vi "Auto.vi"() -> ()   [LabVIEW 2020]
uses:
  Global_Variable/Global.vi
  Global_Variable/A180648.vi
  Global_Variable/System_Conf.vi
  <userlib>/_MGI/1D Array/MGI Running Average/MGI Running Average(DBL).vi
  <userlib>/_MGI/1D Array/MGI Running Average/MGI Running Average(SGL).vi
  Libraries/S7/S7.lvlib
panel:
  out "工位三开始1":u32
  out "工位三开始":u32
  out "工位2开始":u32
  out "用户事件输出":refnum<user-event>
  out "磨合正向初始化":bool
  out "工位三开始计时1":bool
  out "产品变更_Event":refnum<user-event>
  out "NVH":bool=TRUE
  out "T1+T2":dbl
  out "T2":dbl
  out "T1":dbl
  out "吸收电流":sgl
  out "输出扭矩(大)":sgl
  out "输入扭矩":sgl
  out "力特性逆向去程":bool
  out "力特性正向去程":bool
  out "力特性逆向回程":bool
  out "力特性正向回程":bool
  out "工位三开始计时":bool
  out "工位二开始计时":bool
  out "功能正向初始化":bool
  out "功能逆向初始化":bool
  out "空载逆向初始化":bool
  out "空载正向初始化":bool
  out "试验项目":T1(tab)
  out "压装曲线":cluster{dbl[], dbl[]}[](graph)
  out "侧铆曲线":cluster{dbl[], dbl[]}[](graph)
  out "0°曲线":cluster{dbl[], dbl[]}[](graph)
  out "45°曲线":cluster{dbl[], dbl[]}[](graph)
  out "力特性试验":cluster{dbl[], dbl[]}[](graph)
  out "功能试验":cluster{dbl[], dbl[]}[](graph)
  out "电流特性试验":cluster{dbl[], dbl[]}[](graph)
  out "逆向空载试验":cluster{dbl[], dbl[]}[](graph)
  out "磨合":cluster{dbl[], dbl[]}[](graph)
  in  "判定结果":bool[][](array[boolean])=[[TRUE]]
  in  "STEP":string
  # "车速0"
  # "车速1"
  # "车速2"
  # "车速3"
  # "车速4"
  # "车速5"
  # "车速0"
  # "车速1"
  # "车速2"
  # "车速3"
  # "车速4"
  # "车速5"
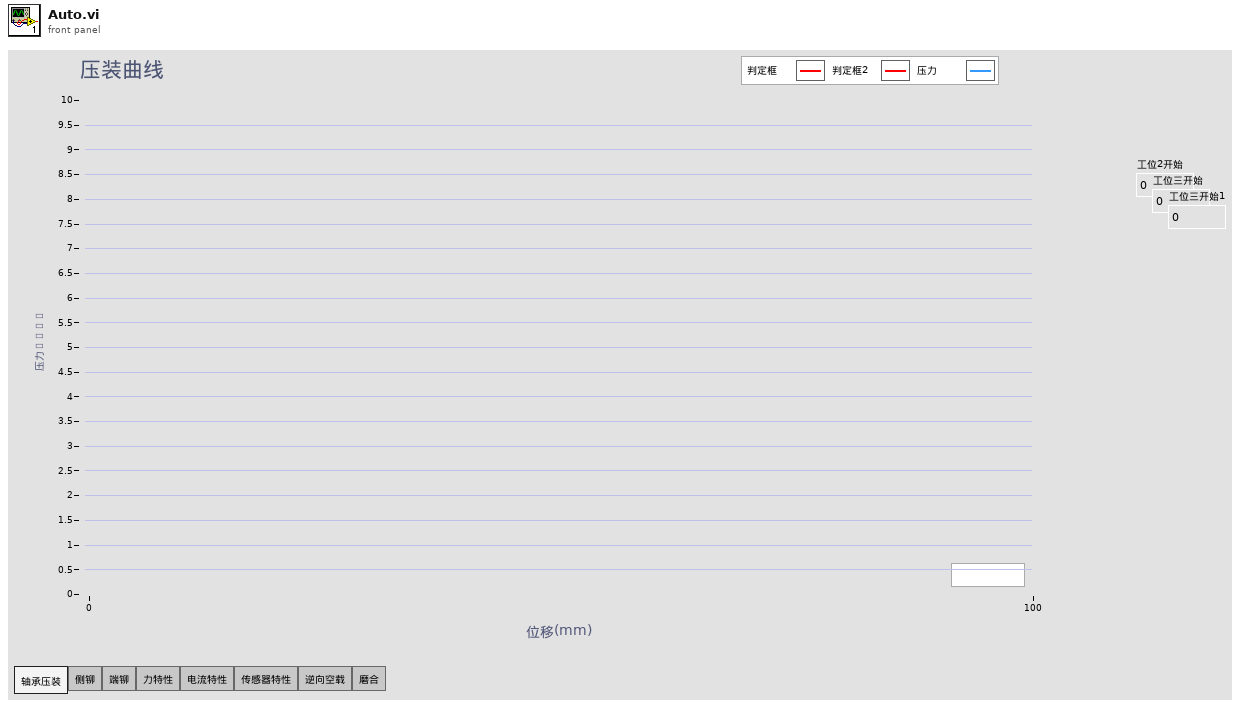
[diagram p1: front panel]
types:
  T1 = enum32{"轴承压装", "侧铆", "端铆", "力特性", "电流特性", "传感器特性", "逆向空载", "磨合"}
  T2 = enum32{"Invalid", "Standard", "Closed", "Hidden", "Minimized", "Maximized"}
  T3 = typedef "lveventtype.ctl" = enum32{"Null", "Timeout", "Annotation Menu Selection", "Annotation Menu Selection?", "App Instance Close", "App Instance Close?", "Autoscale Range Change", "Bookmark Info Change", "Cell Edit", "Cell Edit?", "Cursor Grab", "Cursor Grab?", "Cursor Menu Selection", "Cursor Menu Selection?", "Cursor Move", "Cursor Release", "Data Change", "Direction Change", "Display State Change", "Drag Ended", "Drag Enter", "Drag Leave", "Drag Over", "Drag Source Update", "Drag Starting", "Drag Starting?", "Drop", "Exec State Change", "Key Down", "Key Down?", "Key Repeat", "Key Repeat?", "Key Up", "Listbox Double Click", "Menu Activation?", "Menu Selection (App)", "Menu Selection? (App)", "Menu Selection (User)", "Mouse Down", "Mouse Down?", "Mouse Enter", "Mouse Leave", "Mouse Move", "Mouse Up", "Mouse Wheel", "NI Security User Change (App)", "Pane Size", "Panel Close", "Panel Close?", "Panel Resize", "Plot Attribute Change", "Scale Range Change", "Shortcut Menu Activation?", "Shortcut Menu Selection (App)", "Shortcut Menu Selection? (App)", "Shortcut Menu Selection (User)", "Tree Double Click", "Tree Drag", "Tree Drag?", "Tree Drop", "Tree Drop?", "Tree Item Close", "Tree Item Close?", "Tree Item Open", "Tree Item Open?", "User Event", "Value Change"}
  T4 = typedef "LVPoint32TypeDef.ctl" = cluster{"Horizontal":i32, "Vertical":i32}
  T5 = cluster{"输入轴扭矩":dbl, "输出轴扭矩小量程":dbl, "输出轴扭矩大量程":dbl}
  T6 = typedef "System_conf.ctl" = cluster{"空载滤波":bool, "逆向空载滤波":bool, "空载扭矩系数":dbl, "逆向空载扭矩系数":dbl}
  T7 = cluster{"1位移":cluster{"单位":string, "下限":dbl, "上限":dbl}, "1压力":cluster{"单位":string, "下限":dbl, "上限":dbl}, "2位移":cluster{"单位":string, "下限":dbl, "上限":dbl}, "2压力":cluster{"单位":string, "下限":dbl, "上限":dbl}}
  T8 = cluster{"第一段位移区间最大压力":cluster{"单位":string, "下限":dbl, "上限":dbl}, "第一段位移区间最小压力":cluster{"单位":string, "下限":dbl, "上限":dbl}, "第二段位移区间最大压力":cluster{"单位":string, "下限":dbl, "上限":dbl}, "第二段位移区间最小压力":cluster{"单位":string, "下限":dbl, "上限":dbl}, "压装最终位移":cluster{"单位":string, "下限":dbl, "上限":dbl}}
  T9 = cluster{"侧铆最大压力":cluster{"单位":string, "下限":dbl, "上限":dbl}}
  T10 = cluster{"端铆最大压力":cluster{"单位":string, "下限":dbl, "上限":dbl}}
  T11 = cluster{"端铆0°最大压力":cluster{"单位":string, "下限":dbl, "上限":dbl}, "端铆45°最大压力":cluster{"单位":string, "下限":dbl, "上限":dbl}}
  T12 = cluster{"输入旋转位移":sgl, "输入移载位移":sgl, "工装移载位移":sgl, "备用":sgl, "电缸位移":sgl, "输出扭矩(小)":sgl, "输出扭矩(大)":sgl, "备用1":sgl, "备用2":sgl, "电缸压力":sgl, "2工位压力":sgl, "3工位压力":sgl}
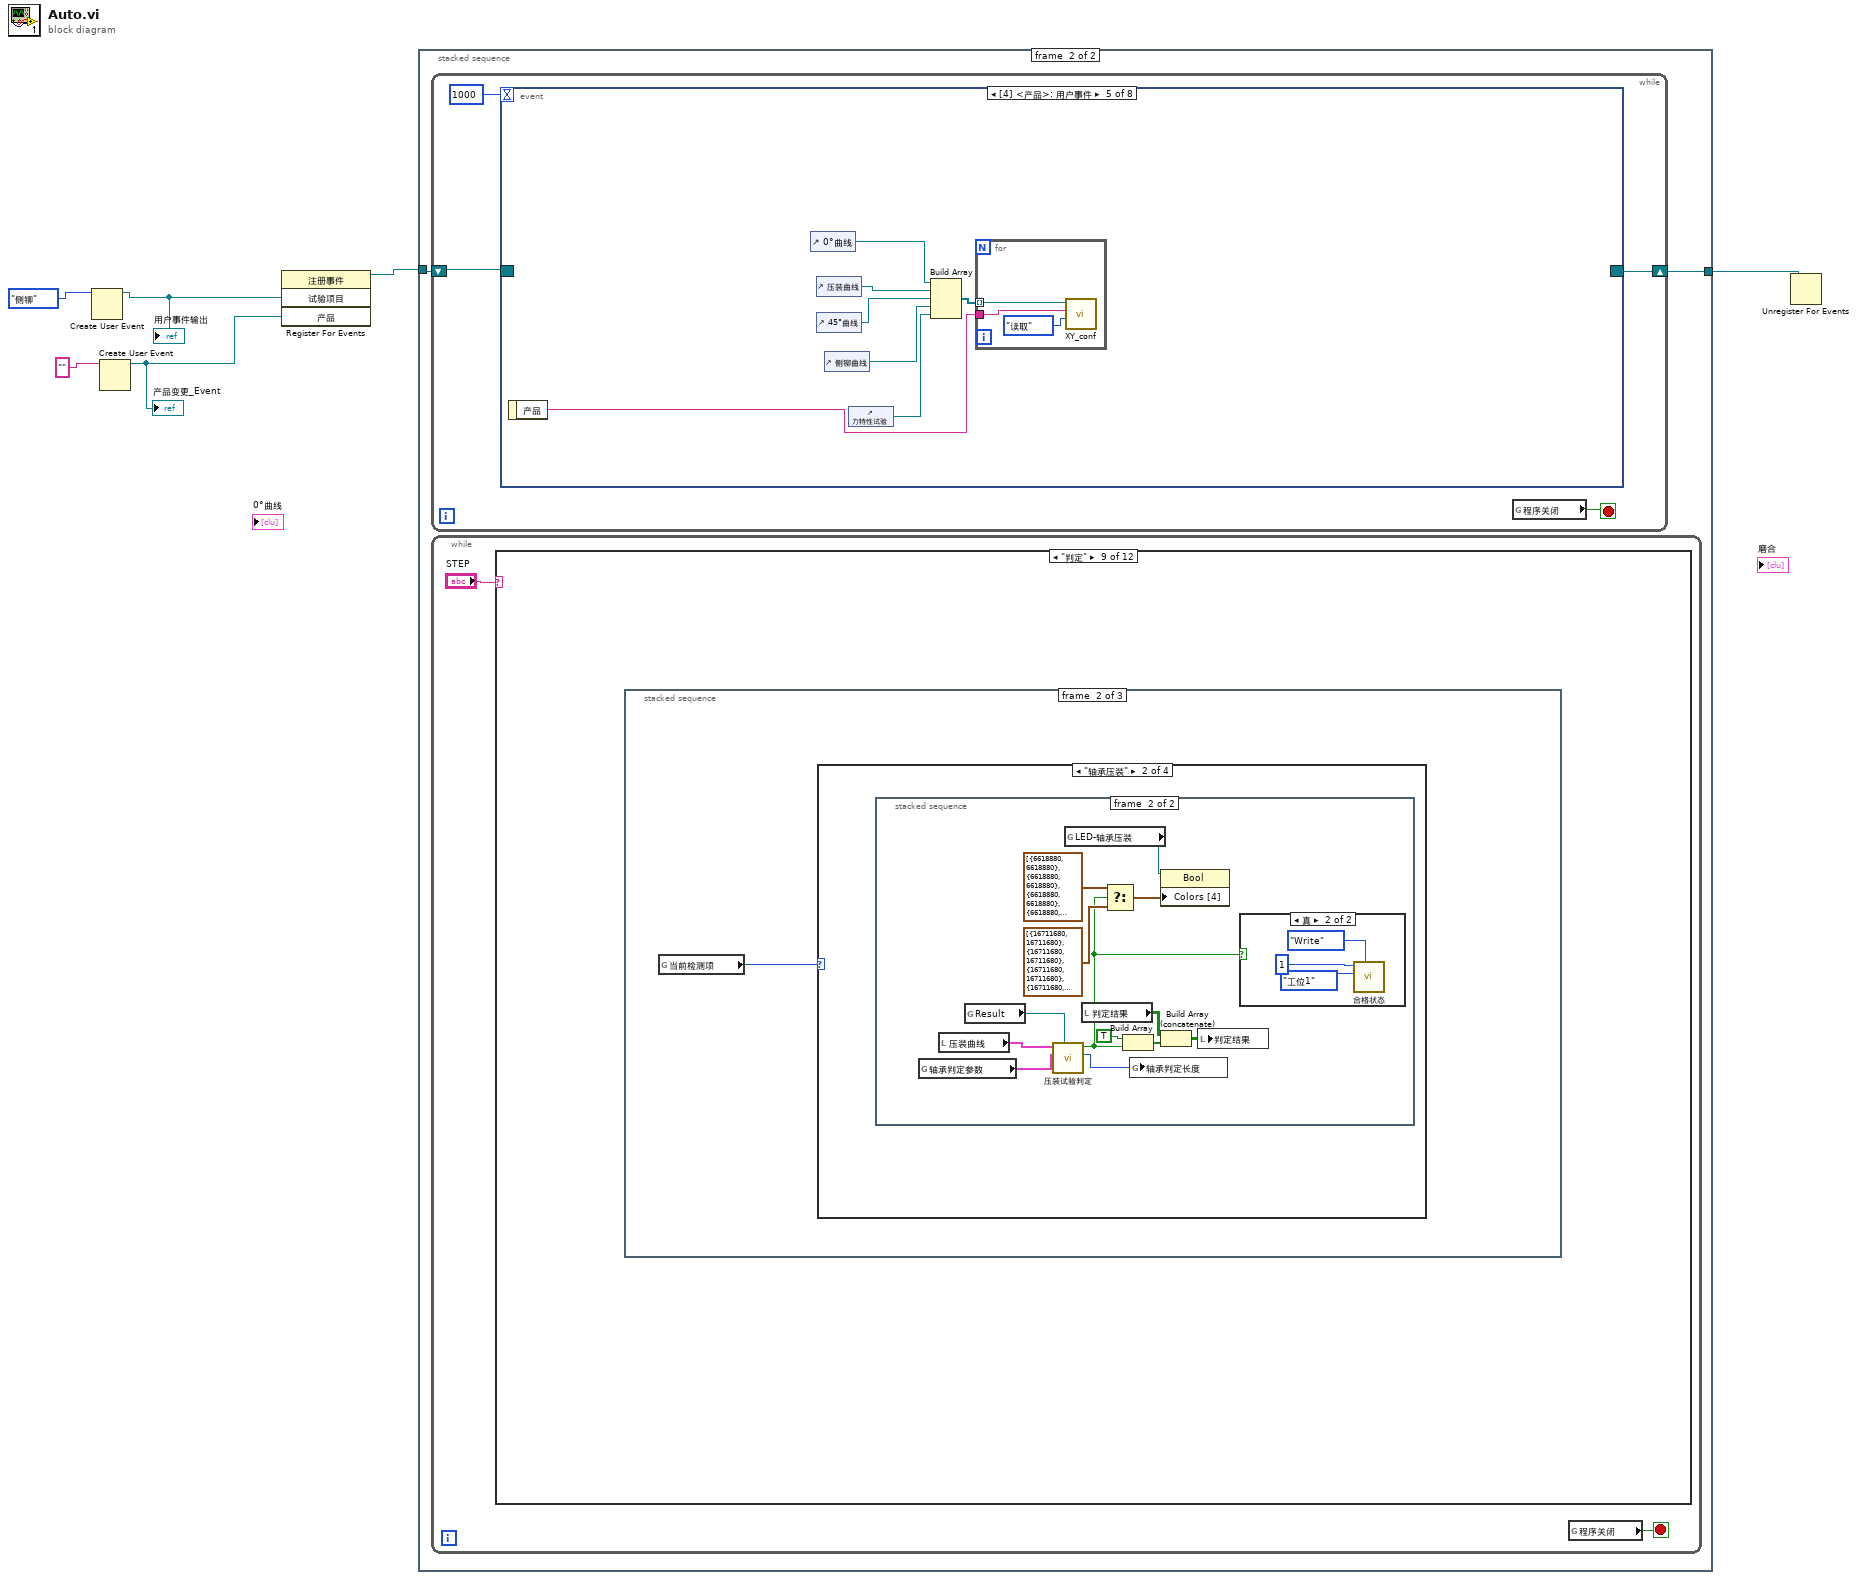
[diagram p0: block diagram]
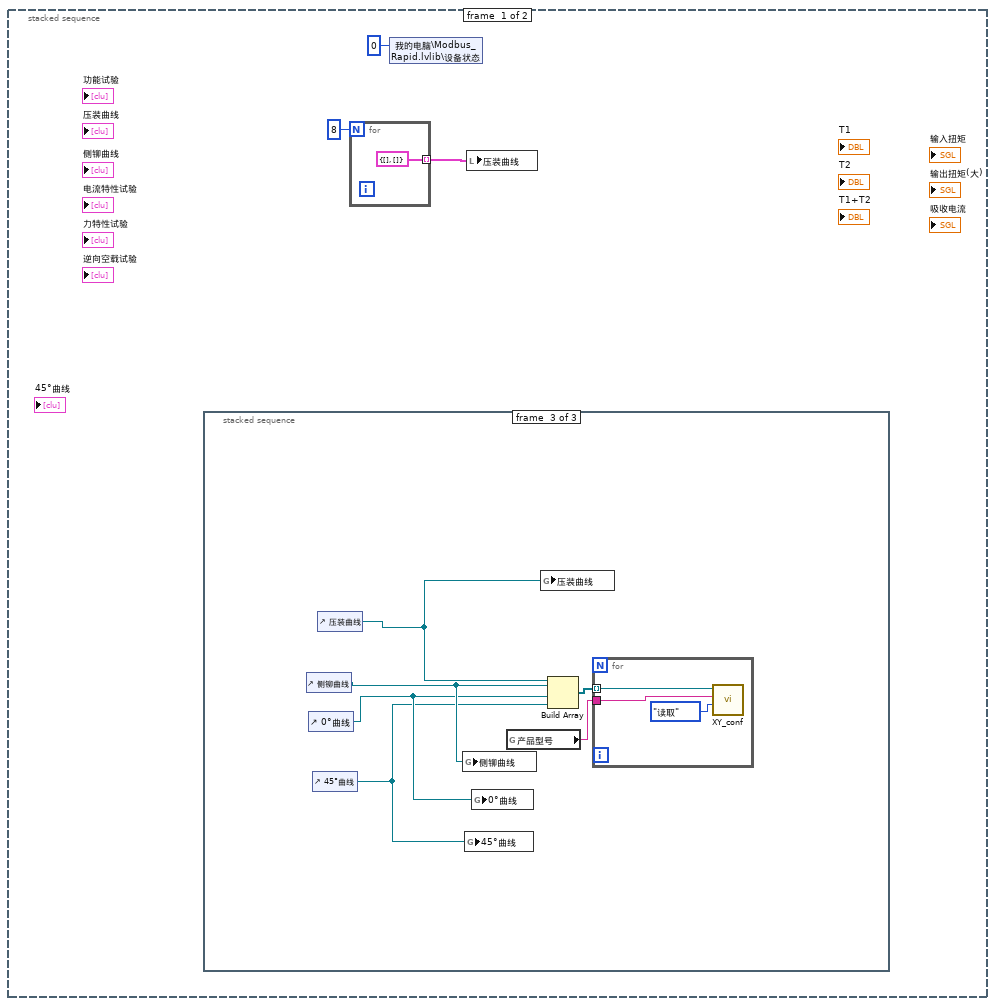
[diagram p2: hidden frame]
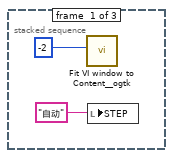
[diagram p3: hidden frame]
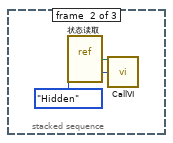
[diagram p4: hidden frame]
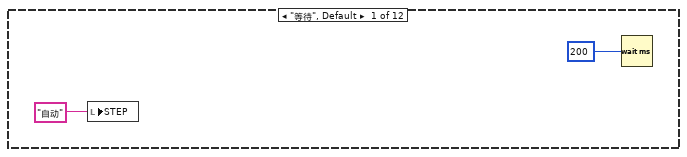
[diagram p5: hidden frame]
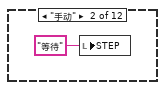
[diagram p6: hidden frame]
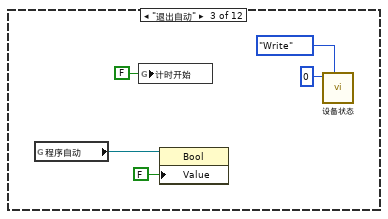
[diagram p7: hidden frame]
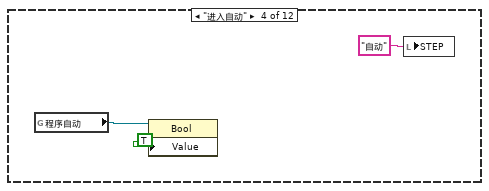
[diagram p8: hidden frame]
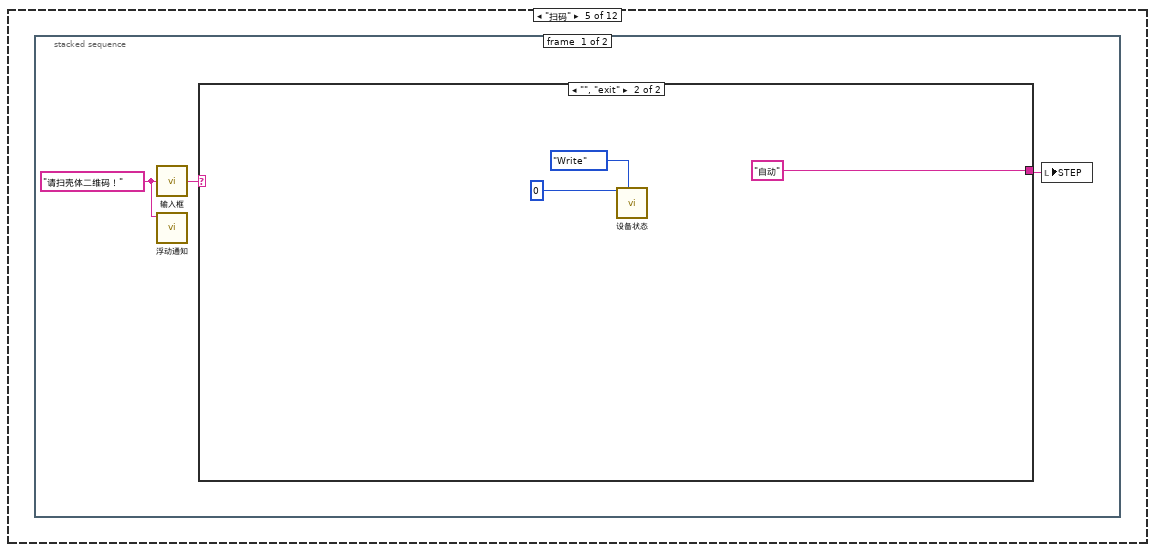
[diagram p9: hidden frame]
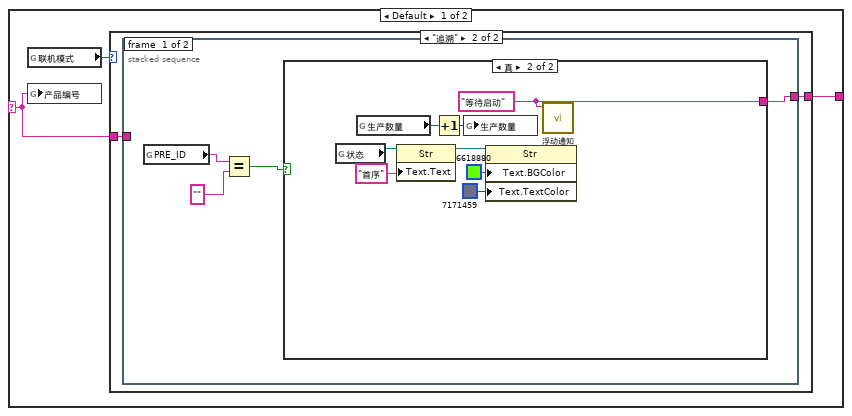
[diagram p10: hidden frame]
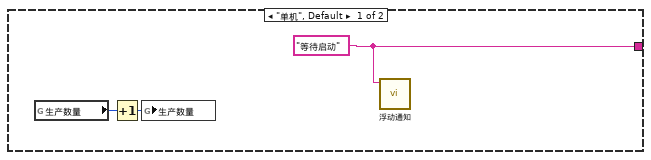
[diagram p11: hidden frame]
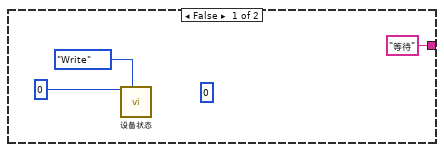
[diagram p12: hidden frame]
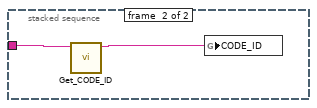
[diagram p13: hidden frame]
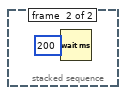
[diagram p14: hidden frame]
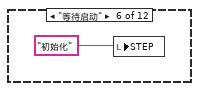
[diagram p15: hidden frame]
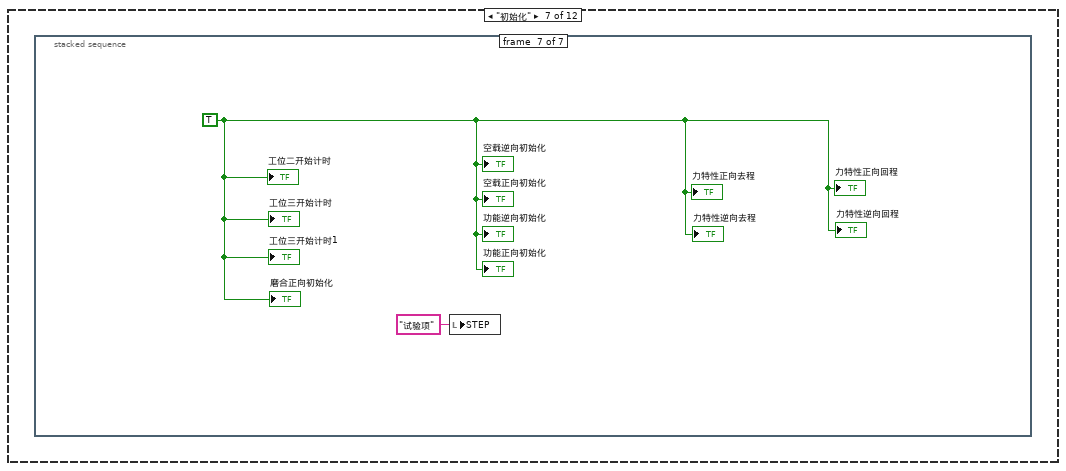
[diagram p16: hidden frame]
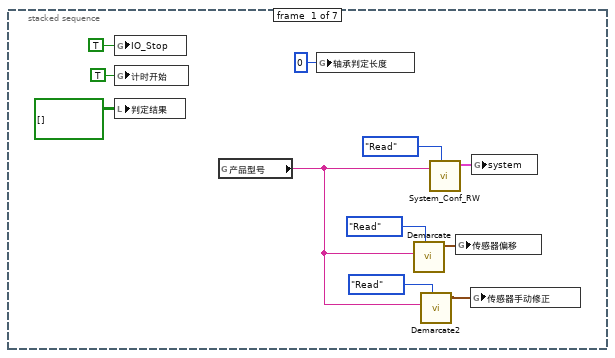
[diagram p17: hidden frame]
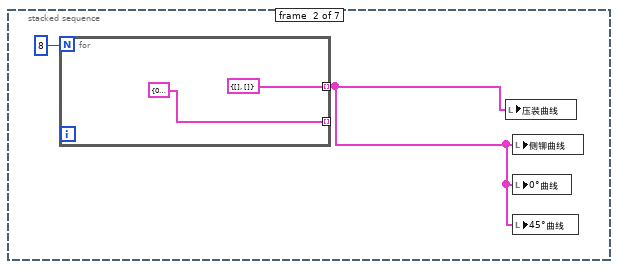
[diagram p18: hidden frame]
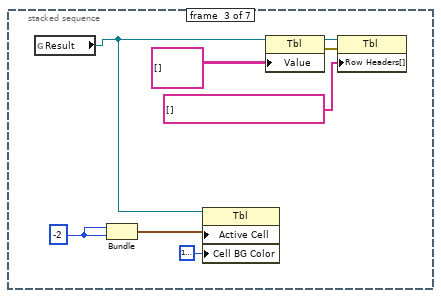
[diagram p19: hidden frame]
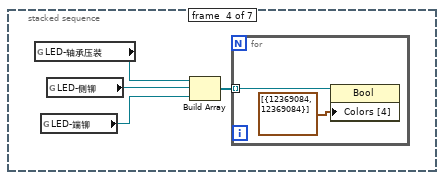
[diagram p20: hidden frame]
diagram:
  n1 = Create User Event(user event datatype=T1."侧铆" ("试验项目")) -> (user event=w1:refnum<user-event>)  [unwired: 1 in, 1 out]
  "用户事件输出" <- w1
  n2 = Create User Event(user event datatype="" ("产品")) -> (user event=w3:refnum<user-event>)  [unwired: 1 in, 1 out]
  "产品变更_Event" <- w3
  n3 = register-events(w1, w3) -> (reference out=w6:refnum<event-registration>)  [unwired: 2 in, 1 out]
  n4 = stacked-sequence {
    tunnel: w6 -> [_ w25]
    tunnel: [_ w24] -> w5
    frame #0 {
      n5 = stacked-sequence {
        frame #0 {
          n6 = call <userlib>:"Fit VI window to Content__ogtk.vi"("border spacing (2 px)"=-2) -> ()  [unwired: 5 in, 2 out]
          n7 = local write "STEP"("自动" ("STEP")) -> ()
        }
        frame #1 {
          n8 = vi-ref "状态读取.vi"() -> (w14:refnum<vi>)
          n9 = call "CallVI.vi"("VI引用"=w14, "状态"=T2."Hidden") -> ()  [unwired: 12 in, 2 out]
        }
        frame #2 {
          n10 = control-ref of="侧铆曲线"() -> (w18:refnum<vi>)
          n11 = control-ref of="0°曲线"() -> (w17:refnum<vi>)
          n12 = control-ref of="45°曲线"() -> (w16:refnum<vi>)
          n13 = control-ref of="压装曲线"() -> (w15:refnum<vi>)
          n14 = global write "A180648.vi" "侧铆曲线"(w18) -> ()
          n15 = global write "A180648.vi" "45°曲线"(w16) -> ()
          n16 = global write "A180648.vi" "0°曲线"(w17) -> ()
          n17 = global read "Global.vi" "产品型号"() -> (w19:string)
          n18 = global write "A180648.vi" "压装曲线"(w15) -> ()
          n19 = Build Array(w15, w18, w17, w16) -> (w20:refnum<vi>[])
          n20 = for {
            tunnel: w20 -> [w22] mode=indexing
            tunnel: w19 -> [w21]
            n21 = call "XY_conf.vi"("方式"=enum16{"写入", "读取"}."读取", "产品"=w21, "XY图引用"=w22) -> ()  [unwired: 4 in, 1 out]
          }
        }
      }
      n22 = for {
        N: 8 -> [_]
        tunnel: [cluster{dbl[], dbl[]} {[], []}] -> w9 mode=indexing
      }
      n23 = shared-variable "我的电脑\\Modbus_Rapid.lvlib\\设备状态"(u16 0 ("设备状态")) -> ()  [unwired: 1 in, 1 out]
      n24 = local write "压装曲线"(w9) -> ()
    }
    frame #1 {
      n25 = while {
        shift-right: [w381] -> w24
        shift-left: w25 -> [w382]
        stop <- w383 stop-if-true
        n26 = event shown="[4] <产品>: 用户事件" {
          selector: w382 -> [_ _ _ _ _ _ _ _]
          dyn-events: [_ _ _ _ _ _ _ _] -> w381
          timeout: 1000 -> [_ _ _ _ _ _ _ _]
          event Timeout {
            n27 = event-data() -> ()  [unwired: 1 in, 3 out]
            n28 = call "Obtain Broadcast Events for Registration.vi"() -> ("Already running?"=w385:bool)  [unwired: 9 in, 2 out]
            n29 = case shown="真" w385 {
              frame False {
                n30 = local write "STEP"("手动" ("STEP")) -> ()
              }
              frame True {
                n31 = call "错误代码.vi"() -> ("Status_Read"=w387:u32)  [unwired: 11 in]
                n32 = feedback #1() -> (w397:u32)  [unwired: 1 in]
                n33 = feedback-in #1(w387) -> ()
                n34 = case shown="0" w387 {
                  frame 0 {
                    n35 = global read "Global.vi" "报警图标"() -> (w398:refnum<vi>)
                    n36 = property class="Bool"(reference=w398, "Visible"=FALSE ("可见")) -> ()  [unwired: 1 in, 2 out]
                  }
                  frame 1, Default {
                    n37 = global read "Global.vi" "报警图标"() -> (w401:refnum<vi>)
                    n38 = property class="Bool"(reference=w401, "Visible"=TRUE ("可见")) -> ()  [unwired: 1 in, 2 out]
                  }
                }
                n39 = Greater Or Equal?(x=w387, y=i16 5000) -> (x >= y?=w395:bool)
                n40 = Less?(x=w387, y=i16 5200) -> (x < y?=w396:bool)
                n41 = Equal?(x=w387, y=w397) -> (x = y?=w394:bool)
                n42 = global read "Global.vi" "报警图标"() -> (w389:refnum<vi>)
                n43 = And(x=w395, y=w396) -> (x .and. y?=w388:bool)
                n44 = property class="Bool"(reference=w389, "Value"=w388) -> ()  [unwired: 1 in, 2 out]
                n45 = Bundle By Name(cluster=errorcluster {"status"=FALSE, "code"=0, "source"=""} ("错误常量"), "status"=w388, "code"=w387) -> (w393:errorcluster)
                n46 = case shown="假" w394 {
                  tunnel: w393 -> [w402 _]
                  frame False {
                    n47 = call "报警处理.vi"("错误常量"=w402) -> ()  [unwired: 9 in, 2 out]
                  }
                  frame True {
                  }
                }
              }
            }
          }
          event User Event {
            n48 = event-data() -> ("试验项目"=w403:T1)  [unwired: 1 in]
            "试验项目" <- w403
            n49 = disable-structure shown="禁用" {
              disable-tunnel: w403 -> [w404 _]
              frame Disabled {
                n50 = global read "A180648.vi" "检测结果"() -> (w407:string[][][])
                n51 = global read "Global.vi" "Result"() -> (w405:refnum<vi>)
                n52 = Index Array(array=w407, index (dim 0)=w404) -> (element=w406:string[][])  [unwired: 2 in]
                n53 = property class="Tbl"(reference=w405, "Value"=w406) -> ()  [unwired: 1 in, 2 out]
              }
              frame Enabled {
              }
            }
          }
          event "试验项目": Value Change {
            n54 = event-data() -> ("NewVal"=w408:T1)  [unwired: 1 in]
            n55 = disable-structure shown="禁用" {
              disable-tunnel: w408 -> [w412 _]
              frame Disabled {
                n56 = global read "A180648.vi" "检测结果"() -> (w411:string[][][])
                n57 = global read "Global.vi" "Result"() -> (w409:refnum<vi>)
                n58 = Index Array(array=w411, index (dim 0)=w412) -> (element=w410:string[][])  [unwired: 2 in]
                n59 = property class="Tbl"(reference=w409, "Value"=w410) -> ()  [unwired: 1 in, 2 out]
              }
              frame Enabled {
              }
            }
          }
          event "0°曲线", "侧铆曲线", "45°曲线", "压装曲线", "功能试验", "逆向空载试验", "磨合": Scale Range Change {
            n60 = event-data() -> ("CtlRef"=w414:refnum<vi>)  [unwired: 1 in, 4 out]
            n61 = global read "Global.vi" "产品型号"() -> (w413:string)
            n62 = call "XY_conf.vi"("方式"=enum16{"写入", "读取"}."写入", "产品"=w413, "XY图引用"=w414) -> ()  [unwired: 4 in, 1 out]
          }
          event User Event {
            n63 = event-data() -> ("产品"=w418:string)  [unwired: 1 in]
            n64 = control-ref of="0°曲线"() -> (w417:refnum<vi>)
            n65 = control-ref of="压装曲线"() -> (w420:refnum<vi>)
            n66 = control-ref of="45°曲线"() -> (w416:refnum<vi>)
            n67 = control-ref of="侧铆曲线"() -> (w422:refnum<vi>)
            n68 = control-ref of="力特性试验"() -> (w421:refnum<vi>)
            n69 = Build Array(w417, w420, w416, w422, w421) -> (w419:refnum<vi>[])
            n70 = for {
              tunnel: w419 -> [w424] mode=indexing
              tunnel: w418 -> [w423]
              n71 = call "XY_conf.vi"("方式"=enum16{"写入", "读取"}."读取", "产品"=w423, "XY图引用"=w424) -> ()  [unwired: 4 in, 1 out]
            }
          }
          event Panel Close {
            n72 = event-data() -> ()  [unwired: 1 in, 4 out]
            n73 = global write "Global.vi" "程序关闭"(TRUE ("程序关闭")) -> ()
          }
          event "0°曲线", "侧铆曲线", "45°曲线", "压装曲线", "功能试验", "逆向空载试验", "磨合": Mouse Enter; "0°曲线", "侧铆曲线", "45°曲线", "压装曲线", "功能试验", "逆向空载试验", "磨合": Mouse Leave; "0°曲线", "侧铆曲线", "45°曲线", "压装曲线", "功能试验", "逆向空载试验": Cursor Move; "磨合": Mouse Move {
            n74 = event-data() -> ("CtlRef"=w429:refnum<vi>, "Type"=w427:T3)  [unwired: 1 in]
            n75 = call "CursorShow.vi"("nameShow"=TRUE, "Type"=w427, "Graph"=w429) -> ()  [unwired: 7 in, 2 out]
          }
          event "0°曲线", "侧铆曲线", "45°曲线", "压装曲线", "功能试验", "逆向空载试验", "磨合": Mouse Down {
            n76 = event-data() -> ("CtlRef"=w434:refnum<vi>, "Coords"=w433:T4, "Type"=w431:T3)  [unwired: 1 in]
            n77 = invoke class="XYGraph (严格)" method="Map Coords To XY"(reference=w434, "Coords"=w433) -> (reference out=w432:refnum<vi>, "XY"=w430:cluster{"X":dbl, "Y":dbl})  [unwired: 5 in, 5 out]
            n78 = call "CursorShow.vi"("游标.游标位置"=w430, "Type"=w431, "Graph"=w432) -> ()  [unwired: 7 in, 2 out]
          }
        }
        n79 = global read "Global.vi" "程序关闭"() -> (w383:bool)
      }
      n80 = while {
        stop <- w27 stop-if-true
        n81 = case shown="\"判定\"" "STEP" {
          frame "等待", Default {
            n82 = local write "STEP"("自动" ("STEP")) -> ()
            n83 = Wait (ms)(milliseconds to wait=u32 200 ("等待时间（毫秒）")) -> ()  [unwired: 1 out]
          }
          frame "手动" {
            n84 = local write "STEP"("等待" ("STEP")) -> ()
          }
          frame "退出自动" {
            n85 = global read "Global.vi" "程序自动"() -> (w32:refnum<vi>)
            n86 = global write "Global.vi" "计时开始"(FALSE ("计时开始")) -> ()
            n87 = property class="Bool"(reference=w32, "Value"=FALSE) -> ()  [unwired: 1 in, 2 out]
            n88 = call "设备状态.vi"("枚举"=enum16{"Read", "Write"}."Write", "Status_Write"=i16 0) -> ()  [unwired: 9 in, 1 out]
          }
          frame "进入自动" {
            n89 = global read "Global.vi" "程序自动"() -> (w37:refnum<vi>)
            n90 = property class="Bool"(reference=w37, "Value"=TRUE) -> ()  [unwired: 1 in, 2 out]
            n91 = local write "STEP"("自动" ("STEP")) -> ()
          }
          frame "扫码" {
            n92 = stacked-sequence {
              frame #0 {
                w40 = "请扫壳体二维码！" ("提示信息")
                n93 = call "输入框.vi"("提示信息"=w40) -> ("条形码输出"=w41:string)
                n94 = call "浮动通知.vi"("通知内容"=w40) -> ()  [unwired: 11 in]
                n95 = case shown="\"\", \"exit\"" w41 {
                  selector: w41 -> [w42 _]
                  tunnel: [w44 "自动" ("State(s) in Front (\"\")")] -> w39
                  frame Default {
                    n96 = global read "Global.vi" "联机模式"() -> (w43:enum16{"单机", "追溯"})
                    n97 = global write "Global.vi" "产品编号"(w42) -> ()
                    n98 = case shown="\"追溯\"" w43 {
                      tunnel: [w45 w49] -> w44
                      tunnel: w42 -> [_ w48]
                      frame "单机", Default {
                        w45 = "等待启动" ("State(s) in Front (\"\")")
                        n99 = global read "Global.vi" "生产数量"() -> (w46:i32)
                        n100 = Increment(x=w46) -> (x+1=w47:i32)
                        n101 = global write "Global.vi" "生产数量"(w47) -> ()
                        n102 = call "浮动通知.vi"("通知内容"=w45) -> ()  [unwired: 11 in]
                      }
                      frame "追溯" {
                        n103 = stacked-sequence {
                          tunnel: [w50 _] -> w49
                          tunnel: w48 -> [_ w66]
                          frame #0 {
                            n104 = global read "追溯Global.vi" "PRE_ID"() -> (w53:string)
                            n105 = Equal?(x=w53, y="") -> (x = y?=w51:bool)
                            n106 = case shown="真" w51 {
                              tunnel: ["等待" ("State(s) in Front (\"\")") w57] -> w50
                              frame False {
                                (unwired) u16 0 ("设备状态")
                                n107 = call "设备状态.vi"("枚举"=enum16{"Read", "Write"}."Write", "Status_Write"=u16 0 ("设备状态")) -> ()  [unwired: 9 in, 1 out]
                              }
                              frame True {
                                w57 = "等待启动" ("State(s) in Front (\"\")")
                                n108 = global read "Global.vi" "状态"() -> (w62:refnum<vi>)
                                n109 = global read "Global.vi" "生产数量"() -> (w63:i32)
                                n110 = property class="Str"(reference=w62, "Text.Text"="首序" ("文本.文本")) -> (reference out=w60:refnum<vi>)  [unwired: 1 in, 1 out]
                                n111 = Increment(x=w63) -> (x+1=w64:i32)
                                n112 = global write "Global.vi" "生产数量"(w64) -> ()
                                n113 = property class="Str"(reference=w60, "Text.BGColor"=u32 6618880 ("文本.文本颜色:背景色"), "Text.TextColor"=u32 7171459 ("文本.文本颜色:文本颜色")) -> ()  [unwired: 1 in, 2 out]
                                n114 = call "浮动通知.vi"("通知内容"=w57) -> ()  [unwired: 11 in]
                              }
                            }
                          }
                          frame #1 {
                            n115 = call "Get_CODE_ID.vi"("CODE_MAIN"=w66) -> ("CODE_ID"=w65:string)  [unwired: 10 in]
                            n116 = global write "追溯Global.vi" "CODE_ID"(w65) -> ()
                          }
                        }
                      }
                    }
                  }
                  frame "", "exit" {
                    n117 = call "设备状态.vi"("枚举"=enum16{"Read", "Write"}."Write", "Status_Write"=u16 0 ("设备状态")) -> ()  [unwired: 9 in, 1 out]
                  }
                }
                n118 = local write "STEP"(w39) -> ()
              }
              frame #1 {
                n119 = Wait (ms)(milliseconds to wait=u32 200 ("等待时间（毫秒）")) -> ()  [unwired: 1 out]
              }
            }
          }
          frame "等待启动" {
            n120 = local write "STEP"("初始化" ("STEP")) -> ()
          }
          frame "初始化" {
            n121 = stacked-sequence {
              frame #0 {
                n122 = global write "Global.vi" "IO_Stop"(TRUE ("IO_Stop")) -> ()
                n123 = global write "Global.vi" "计时开始"(TRUE ("计时开始")) -> ()
                n124 = local write "判定结果"(bool[][] [] ("判定结果")) -> ()
                n125 = global read "Global.vi" "产品型号"() -> (w73:string)
                n126 = global write "判定参数.vi" "轴承判定长度"(0 ("轴承判定长度")) -> ()
                n127 = call "Demarcate.vi"("Mode"=enum16{"Read", "Write"}."Read", "Section"=w73) -> ("Sensor OUT"=w77:T5)  [unwired: 8 in, 1 out]
                n128 = call "Demarcate2.vi"("Mode"=enum16{"Read", "Write"}."Read", "Section"=w73) -> ("Sensor OUT"=w76:T5)  [unwired: 8 in, 1 out]
                n129 = call "System_Conf_RW.vi"("Mode"=enum16{"Read", "Write"}."Read", "Section"=w73) -> ("system_out"=w79:T6)  [unwired: 8 in, 1 out]
                n130 = global write "传感器偏移.vi" "传感器偏移"(w77) -> ()
                n131 = global write "传感器偏移.vi" "传感器手动修正"(w76) -> ()
                n132 = global write "System_Conf.vi" "system"(w79) -> ()
              }
              frame #1 {
                n133 = for {
                  N: 8 -> [_]
                  tunnel: [cluster{dbl[], dbl[]} {[], []}] -> w83 mode=indexing
                  tunnel: [cluster{"f0":dbl, "df":dbl, "magnitude":dbl[]} {"f0"=0.0, "df"=0.0, "magnitude"=[]} ("power spectrum [dB EU]")] -> _ mode=indexing
                }
                n134 = local write "压装曲线"(w83) -> ()
                n135 = local write "侧铆曲线"(w83) -> ()
                n136 = local write "0°曲线"(w83) -> ()
                n137 = local write "45°曲线"(w83) -> ()
              }
              frame #2 {
                w88 = -2
                n138 = global read "Global.vi" "Result"() -> (w90:refnum<vi>)
                n139 = Bundle(w88, w88) -> (w87:cluster{i32, i32})  [unwired: 1 in]
                n140 = property class="Tbl"(reference=w90, "Active Cell"=w87, "Cell BG Color"=u32 16777216 ("活动单元格:单元格背景色")) -> ()  [unwired: 1 in, 2 out]
                n141 = property class="Tbl"(reference=w90, "Value"=string[][] []) -> (reference out=w93:refnum<vi>, error out=w94:errorcluster)  [unwired: 1 in]
                n142 = property class="Tbl"(reference=w93, error in=w94, "Row Headers[]"=string[] [] ("列首字符串[]")) -> ()  [unwired: 2 out]
              }
              frame #3 {
                n143 = global read "A180648.vi" "LED-轴承压装"() -> (w98:refnum<vi>)
                n144 = global read "A180648.vi" "LED-端铆"() -> (w95:refnum<vi>)
                n145 = global read "A180648.vi" "LED-侧铆"() -> (w96:refnum<vi>)
                n146 = Build Array(w98, w96, w95) -> (w97:refnum<vi>[])
                n147 = for {
                  tunnel: w97 -> [w99] mode=indexing
                  n148 = property class="Bool"(reference=w99, "Colors [4]"=cluster{u32, u32}[] [{12369084, 12369084}] ("颜色[4]")) -> ()  [unwired: 1 in, 2 out]
                }
              }
              frame #4 {
                w102 = 1 ("维数大小")
                n149 = Initialize Array(" " ("字符串"), w102, w102, w102) -> (w104:string[][][])
                n150 = global write "A180648.vi" "当前检测项"(enum32{"轴承压装", "侧铆", "端铆", "完成"}."轴承压装" ("当前检测项")) -> ()
                n151 = global write "A180648.vi" "检测结果"(w104) -> ()
              }
              frame #5 {
                n152 = local read "压装曲线"() -> (w106:cluster{dbl[], dbl[]}[])
                n153 = global read "判定参数.vi" "判定框"() -> (w107:T7)
                n154 = for {
                  tunnel: w106 -> [w110] mode=indexing
                  tunnel: [w109] -> w105 mode=indexing
                  tunnel: w107 -> [w108]
                  i -> [w111]
                  n155 = case shown="0" w111 {
                    tunnel: w110 -> [w112 _ _]
                    tunnel: [w112 w115 w123] -> w109
                    tunnel: w108 -> [_ w120 w124]
                    frame Default {
                    }
                    frame 0 {
                      n156 = Unbundle By Name(w120) -> ("1位移.下限"=w119:dbl, "1位移.上限"=w118:dbl, "1压力.下限"=w113:dbl, "1压力.上限"=w114:dbl)
                      n157 = Build Array(w118, w118, w119, w119, w118) -> (w117:dbl[])
                      n158 = Build Array(w113, w114, w114, w113, w113) -> (w116:dbl[])
                      n159 = Bundle(w117, w116) -> (w115:cluster{dbl[], dbl[]})  [unwired: 1 in]
                    }
                    frame 1 {
                      n160 = Unbundle By Name(w124) -> ("2位移.下限"=w128:dbl, "2位移.上限"=w127:dbl, "2压力.下限"=w121:dbl, "2压力.上限"=w122:dbl)
                      n161 = Build Array(w127, w127, w128, w128, w127) -> (w126:dbl[])
                      n162 = Build Array(w121, w122, w122, w121, w121) -> (w125:dbl[])
                      n163 = Bundle(w126, w125) -> (w123:cluster{dbl[], dbl[]})  [unwired: 1 in]
                    }
                  }
                }
                n164 = local write "压装曲线"(w105) -> ()
              }
              frame #6 {
                w130 = TRUE
                n165 = local write "STEP"("试验项" ("STEP")) -> ()
                "工位三开始计时" <- w130
                "工位二开始计时" <- w130
                "空载正向初始化" <- w130
                "空载逆向初始化" <- w130
                "功能正向初始化" <- w130
                "功能逆向初始化" <- w130
                "力特性逆向去程" <- w130
                "力特性正向去程" <- w130
                "力特性逆向回程" <- w130
                "力特性正向回程" <- w130
                "磨合正向初始化" <- w130
                "工位三开始计时1" <- w130
              }
            }
          }
          frame "试验项" {
            n166 = global read "A180648.vi" "当前检测项"() -> (w131:enum32{"轴承压装", "侧铆", "端铆", "完成"})
            n167 = case shown="\"轴承压装\", 默认" w131 {
              selector: w131 -> [w133 _]
              tunnel: [w136 "报表" ("STEP")] -> w132
              frame "轴承压装", Default {
                n168 = global read "Global.vi" "试验项目"() -> (w134:bool[])
                n169 = Index Array(array=w134, index=w133) -> (element=w135:bool)
                n170 = case shown="真" w135 {
                  tunnel: ["试验项" ("字符串") w143] -> w136
                  tunnel: w133 -> [_ w144]
                  frame False {
                    n171 = global read "A180648.vi" "当前检测项"() -> (w141:enum32{"轴承压装", "侧铆", "端铆", "完成"})
                    n172 = Increment(x=w141) -> (x+1=w140:enum32{"轴承压装", "侧铆", "端铆", "完成"})
                    n173 = global write "A180648.vi" "当前检测项"(w140) -> ()
                    n174 = local read "判定结果"() -> (w137:bool[][])
                    n175 = Build Array (concatenate)(w137, bool[] [FALSE] ("判定结果")) -> (w138:bool[][])
                    n176 = local write "判定结果"(w138) -> ()
                  }
                  frame True {
                    n177 = case shown="\"轴承压装\", 默认" w144 {
                      tunnel: ["等待" ("STEP") "等待" ("STEP") "等待" ("STEP")] -> w143
                      frame "轴承压装", Default {
                        n178 = call "浮动通知.vi"("通知内容"="轴承压装") -> ()  [unwired: 11 in]
                        n179 = property on="试验项目" class="TabCtl (严格)"("Val(Sgnl)"=T1."轴承压装" ("值(信号)")) -> ()  [unwired: 2 in, 2 out]
                        n180 = call "设备状态.vi"("枚举"=enum16{"Read", "Write"}."Write", "Status_Write"=u16 1002 ("设备状态")) -> ()  [unwired: 9 in, 1 out]
                        n181 = Wait Until Next ms Multiple(millisecond multiple=u32 100 ("毫秒倍数")) -> ()  [unwired: 1 out]
                      }
                      frame "侧铆" {
                        n182 = call "浮动通知.vi"("通知内容"="侧铆") -> ()  [unwired: 11 in]
                      }
                      frame "端铆" {
                        n183 = call "浮动通知.vi"("通知内容"="端铆") -> ()  [unwired: 11 in]
                      }
                    }
                  }
                }
              }
              frame "完成" {
              }
            }
            n184 = local write "STEP"(w132) -> ()
          }
          frame "判定" {
            n185 = stacked-sequence {
              frame #0 {
                n186 = call "设备状态.vi"("枚举"=enum16{"Read", "Write"}."Write", "Status_Write"=u16 0 ("设备状态")) -> ()  [unwired: 9 in, 1 out]
              }
              frame #1 {
                n187 = global read "A180648.vi" "当前检测项"() -> (w158:enum32{"轴承压装", "侧铆", "端铆", "完成"})
                n188 = case shown="\"轴承压装\"" w158 {
                  frame "完成", Default {
                  }
                  frame "轴承压装" {
                    n189 = stacked-sequence {
                      frame #0 {
                        n190 = global read "Global.vi" "联机模式"() -> (w159:enum16{"单机", "追溯"})
                        n191 = case shown="\"追溯\"" w159 {
                          frame "单机", Default {
                          }
                          frame "追溯" {
                            n192 = global read "追溯Global.vi" "PRODUCT_ID"() -> (w160:string)
                            n193 = global read "Global.vi" "产品编号"() -> (w161:string)
                            n194 = call "INTOCODE.vi"("CODE_MAIN"=w161, "PRODUCT_ID"=w160) -> ()  [unwired: 13 in, 1 out]
                          }
                        }
                      }
                      frame #1 {
                        n195 = global read "判定参数.vi" "轴承判定参数"() -> (w173:T8)
                        n196 = local read "压装曲线"() -> (w174:cluster{dbl[], dbl[]}[])
                        n197 = global read "Global.vi" "Result"() -> (w172:refnum<vi>)
                        n198 = call "压装试验判定.vi"("Result"=w172, "判定参数"=w173, "XY曲线"=w174) -> ("判定项长度"=w163:i32, "OK？"=w162:bool)  [unwired: 7 in]
                        n199 = global read "A180648.vi" "LED-轴承压装"() -> (w168:refnum<vi>)
                        n200 = local read "判定结果"() -> (w164:bool[][])
                        n201 = Select(t=cluster{u32, u32}[] [{6618880, 6618880}, {6618880, 6618880}, {6618880, 6618880}, {6618880, 6618880}] ("颜色[4]"), s=w162, f=cluster{u32, u32}[] [{16711680, 16711680}, {16711680, 16711680}, {16711680, 16711680}, {16711680, 16711680}] ("颜色[4]")) -> (s? t:f=w169:cluster{u32, u32}[])
                        n202 = Build Array(TRUE, w162) -> (w167:bool[])
                        n203 = global write "判定参数.vi" "轴承判定长度"(w163) -> ()
                        n204 = property class="Bool"(reference=w168, "Colors [4]"=w169) -> ()  [unwired: 1 in, 2 out]
                        n205 = Build Array (concatenate)(w164, w167) -> (w165:bool[][])
                        n206 = local write "判定结果"(w165) -> ()
                        n207 = case shown="真" w162 {
                          frame False {
                            n208 = call "合格状态.vi"("枚举"=enum16{"Read", "Write"}."Write", "工位"=enum16{"工位1", "工位2", "工位3"}."工位1", "Status_Write"=u16 2 ("侧铆合格状态")) -> ()  [unwired: 8 in, 1 out]
                          }
                          frame True {
                            n209 = call "合格状态.vi"("枚举"=enum16{"Read", "Write"}."Write", "工位"=enum16{"工位1", "工位2", "工位3"}."工位1", "Status_Write"=u16 1 ("侧铆合格状态")) -> ()  [unwired: 8 in, 1 out]
                          }
                        }
                      }
                    }
                  }
                  frame "侧铆" {
                    n210 = global read "判定参数.vi" "侧铆判定参数"() -> (w193:T9)
                    n211 = local read "侧铆曲线"() -> (w194:cluster{dbl[], dbl[]}[])
                    n212 = global read "Global.vi" "Result"() -> (w192:refnum<vi>)
                    n213 = call "侧铆试验判定.vi"("Result"=w192, "判定参数"=w193, "XY曲线"=w194) -> ("判定项长度"=w183:i32, "OK？"=w181:bool)  [unwired: 7 in]
                    n214 = global read "A180648.vi" "LED-侧铆"() -> (w188:refnum<vi>)
                    n215 = local read "判定结果"() -> (w184:bool[][])
                    n216 = Select(t=cluster{u32, u32}[] [{6618880, 6618880}, {6618880, 6618880}, {6618880, 6618880}, {6618880, 6618880}] ("颜色[4]"), s=w181, f=cluster{u32, u32}[] [{16711680, 16711680}, {16711680, 16711680}, {16711680, 16711680}, {16711680, 16711680}] ("颜色[4]")) -> (s? t:f=w189:cluster{u32, u32}[])
                    n217 = Build Array(TRUE, w181) -> (w187:bool[])
                    n218 = global write "判定参数.vi" "侧铆判定长度"(w183) -> ()
                    n219 = property class="Bool"(reference=w188, "Colors [4]"=w189) -> ()  [unwired: 1 in, 2 out]
                    n220 = Build Array (concatenate)(w184, w187) -> (w185:bool[][])
                    n221 = case shown="假" w181 {
                      frame False {
                        n222 = call "合格状态.vi"("枚举"=enum16{"Read", "Write"}."Write", "工位"=enum16{"工位1", "工位2", "工位3"}."工位3", "Status_Write"=u16 2 ("侧铆合格状态")) -> ()  [unwired: 8 in, 1 out]
                      }
                      frame True {
                        n223 = call "合格状态.vi"("枚举"=enum16{"Read", "Write"}."Write", "工位"=enum16{"工位1", "工位2", "工位3"}."工位3", "Status_Write"=u16 1 ("侧铆合格状态")) -> ()  [unwired: 8 in, 1 out]
                      }
                    }
                    n224 = local write "判定结果"(w185) -> ()
                    "NVH" <- TRUE
                  }
                  frame "端铆" {
                    n225 = global read "Global.vi" "八点"() -> (w202:bool)
                    n226 = local read "45°曲线"() -> (w201:cluster{dbl[], dbl[]}[])
                    n227 = global read "Global.vi" "Result"() -> (w204:refnum<vi>)
                    n228 = case shown="真" w202 {
                      tunnel: [w217 w224] -> w205
                      tunnel: w204 -> [w215 w223]
                      tunnel: [w216 w220] -> w203
                      tunnel: w201 -> [w218 w219]
                      frame False {
                        n229 = global read "判定参数.vi" "八点端铆判定参数"() -> (w214:T10)
                        n230 = call "8点端铆试验判定.vi"("Result"=w215, "判定参数"=w214, "XY曲线 2"=w218) -> ("判定项长度"=w217:i32, "OK？"=w216:bool)  [unwired: 7 in]
                      }
                      frame True {
                        n231 = global read "判定参数.vi" "端铆判定参数"() -> (w221:T11)
                        n232 = local read "0°曲线"() -> (w222:cluster{dbl[], dbl[]}[])
                        n233 = call "端铆试验判定.vi"("Result"=w223, "判定参数"=w221, "XY曲线 2"=w219, "XY曲线"=w222) -> ("判定项长度"=w224:i32, "OK？"=w220:bool)  [unwired: 6 in]
                      }
                    }
                    n234 = global read "A180648.vi" "LED-端铆"() -> (w212:refnum<vi>)
                    n235 = local read "判定结果"() -> (w206:bool[][])
                    n236 = global write "判定参数.vi" "端铆判定长度"(w205) -> ()
                    n237 = Select(t=cluster{u32, u32}[] [{6618880, 6618880}, {6618880, 6618880}, {6618880, 6618880}, {6618880, 6618880}] ("颜色[4]"), s=w203, f=cluster{u32, u32}[] [{16711680, 16711680}, {16711680, 16711680}, {16711680, 16711680}, {16711680, 16711680}] ("颜色[4]")) -> (s? t:f=w213:cluster{u32, u32}[])
                    n238 = Build Array(TRUE, w203) -> (w209:bool[])
                    n239 = case shown="真" w203 {
                      frame False {
                        n240 = call "合格状态.vi"("枚举"=enum16{"Read", "Write"}."Write", "工位"=enum16{"工位1", "工位2", "工位3"}."工位3", "Status_Write"=u16 2 ("侧铆合格状态")) -> ()  [unwired: 8 in, 1 out]
                      }
                      frame True {
                        n241 = call "合格状态.vi"("枚举"=enum16{"Read", "Write"}."Write", "工位"=enum16{"工位1", "工位2", "工位3"}."工位3", "Status_Write"=u16 1 ("侧铆合格状态")) -> ()  [unwired: 8 in, 1 out]
                      }
                    }
                    n242 = property class="Bool"(reference=w212, "Colors [4]"=w213) -> ()  [unwired: 1 in, 2 out]
                    n243 = Build Array (concatenate)(w206, w209) -> (w207:bool[][])
                    n244 = local write "判定结果"(w207) -> ()
                  }
                }
              }
              frame #2 {
                n245 = call "合格状态.vi"("枚举"=enum16{"Read", "Write"}."Read", "工位"=enum16{"工位1", "工位2", "工位3"}."工位1", "Status_Write"=u16 2 ("侧铆合格状态")) -> ("Status_Read"=w231:i16)  [unwired: 8 in]
                n246 = case shown="1, 默认" w231 {
                  frame 1, Default {
                    n247 = global read "A180648.vi" "当前检测项"() -> (w236:enum32{"轴承压装", "侧铆", "端铆", "完成"})
                    n248 = Increment(x=w236) -> (x+1=w237:enum32{"轴承压装", "侧铆", "端铆", "完成"})
                    n249 = global write "A180648.vi" "当前检测项"(w237) -> ()
                    n250 = local write "STEP"("试验项" ("STEP")) -> ()
                  }
                  frame 2 {
                    n251 = local write "STEP"("报表" ("STEP")) -> ()
                  }
                }
              }
            }
          }
          frame "自动" {
            n252 = global read "Global.vi" "设备状态"() -> (w239:i16)
            n253 = case shown="999" w239 {
              frame -128 {
                n254 = global write "Global.vi" "计时开始"(FALSE ("计时开始")) -> ()
                n255 = call "浮动通知.vi"("通知内容"="复位中……" ("Status")) -> ()  [unwired: 11 in]
              }
              frame Default {
              }
              frame 0 {
                n256 = disable-structure shown="禁用" {
                  frame Disabled {
                    n257 = global write "Global.vi" "计时开始"(FALSE ("计时开始")) -> ()
                  }
                  frame Enabled {
                  }
                }
              }
              frame 1 {
                n258 = call "传感器数据.vi"() -> ("传感器读数"=w245:T12)  [unwired: 11 in]
                n259 = Unbundle By Name(w245) -> ("电缸位移"=w244:sgl, "电缸压力"=w243:sgl)
                n260 = disable-structure shown="禁用" {
                  frame Disabled {
                    n261 = local read "压装曲线"() -> (w248:cluster{dbl[], dbl[]}[])
                    n262 = for {
                      tunnel: [w250] -> _ mode=indexing
                      tunnel: w248 -> [w249] mode=indexing
                      i -> [w251]
                      n263 = case shown="2" w251 {
                        tunnel: [_ w252] -> w250
                        tunnel: w249 -> [_ w257]
                        frame Default {
                        }
                        frame 2 {
                          n264 = Unbundle(w257) -> (w256:dbl[], w255:dbl[])
                          n265 = Build Array(w256) -> (w254:dbl[][])  [unwired: 1 in]
                          n266 = Build Array(w255) -> (w253:dbl[][])  [unwired: 1 in]
                          n267 = Bundle(w254, w253) -> (w252:cluster{dbl[][], dbl[][]})  [unwired: 1 in]
                        }
                      }
                    }
                    n268 = local read "压装曲线"() -> ()  [unwired: 1 in]
                  }
                  frame Enabled {
                  }
                }
                n269 = control-ref of="压装曲线"() -> (w247:refnum<vi>)
                n270 = call "曲线采集.vi"("曲线引用"=w247, "曲线索引"=2, "X"=w244, "Y"=w243) -> ()  [unwired: 10 in, 2 out]
              }
              frame 2 {
                n271 = local write "STEP"("判定" ("STEP")) -> ()
              }
              frame 5 {
                n272 = global write "A180648.vi" "当前检测项"(enum32{"轴承压装", "侧铆", "端铆", "完成"}."侧铆" ("当前检测项")) -> ()
                n273 = local write "STEP"("试验项" ("STEP")) -> ()
              }
              frame 3 {
                n274 = global write "A180648.vi" "当前检测项"(enum32{"轴承压装", "侧铆", "端铆", "完成"}."端铆" ("当前检测项")) -> ()
                n275 = local write "STEP"("试验项" ("STEP")) -> ()
              }
              frame 8 {
                n276 = call "浮动通知.vi"("通知内容"="程序停止！" ("Status")) -> ()  [unwired: 11 in]
              }
              frame 10 {
                n277 = local write "STEP"("判定" ("STEP")) -> ()
              }
              frame 30 {
                n278 = local write "STEP"("判定" ("STEP")) -> ()
              }
              frame 100 {
                n279 = local write "STEP"("报表" ("STEP")) -> ()
              }
              frame 114 {
                n280 = global read "System_Conf.vi" "system"() -> (w271:T6)
                n281 = call "传感器数据.vi"() -> ("传感器读数"=w278:T12)  [unwired: 11 in]
                n282 = Unbundle By Name(w278) -> ("输入旋转位移"=w277:sgl, "电缸位移"=w276:sgl)
                n283 = Unbundle By Name(w271) -> ("空载滤波"=w270:bool, "空载扭矩系数"=w268:dbl)
                n284 = local read "空载逆向初始化"() -> (w267:bool)
                n285 = Multiply(x=w276, y=w268) -> (x*y=w269:dbl)
                n286 = case shown="真" w270 {
                  tunnel: w277 -> [w282 w288]
                  tunnel: w269 -> [w281 w287]
                  tunnel: [w282 w285] -> w275
                  tunnel: [w281 w284] -> w274
                  tunnel: w267 -> [_ w283]
                  frame False {
                  }
                  frame True {
                    w286 = 10 ("Averaging Size")
                    n287 = call-poly <userlib>:"MGI Running Average.vi"("Averaging Size"=w286, "Initialize? (F)"=w283, "Value"=w288) -> ("Average"=w285:sgl)  [unwired: 8 in]
                    n288 = call-poly <userlib>:"MGI Running Average.vi"("Averaging Size"=w286, "Initialize? (F)"=w283, "Value"=w287) -> ("Average"=w284:dbl)  [unwired: 8 in]
                  }
                }
                n289 = control-ref of="压装曲线"() -> (w280:refnum<vi>)
                n290 = call "曲线采集.vi"("曲线引用"=w280, "曲线索引"=1, "X"=w275, "Y"=w274) -> ("错误输出"=w273:errorcluster)  [unwired: 10 in, 1 out]
                n291 = Unbundle By Name(w273) -> ("status"=w272:bool)
                n292 = local write "空载逆向初始化"(w272) -> ()
              }
              frame 124 {
                w294 = 1 ("Averaging Size")
                n293 = control-ref of="功能试验"() -> (w292:refnum<vi>)
                n294 = call "传感器数据.vi"() -> ("传感器读数"=w302:T12)  [unwired: 11 in]
                n295 = local read "功能逆向初始化"() -> (w295:bool)
                n296 = Unbundle By Name(w302) -> ("输入旋转位移"=w301:sgl, "电缸位移"=w299:sgl, "输出扭矩(大)"=w297:sgl)
                n297 = call-poly <userlib>:"MGI Running Average.vi"("Averaging Size"=w294, "Initialize? (F)"=w295, "Value"=w299) -> ("Average"=w298:sgl)  [unwired: 8 in]
                n298 = call-poly <userlib>:"MGI Running Average.vi"("Averaging Size"=w294, "Initialize? (F)"=w295, "Value"=w297) -> ("Average"=w296:sgl)  [unwired: 8 in]
                n299 = call-poly <userlib>:"MGI Running Average.vi"("Averaging Size"=w294, "Initialize? (F)"=w295, "Value"=w301) -> ("Average"=w300:sgl)  [unwired: 8 in]
                n300 = call "曲线采集.vi"("曲线引用"=w292, "曲线索引"=1, "X"=w300, "Y"=w298) -> ("错误输出"=w290:errorcluster)  [unwired: 10 in, 1 out]
                n301 = call "曲线采集.vi"("曲线引用"=w292, "曲线索引"=3, "X"=w300, "Y"=w296) -> ()  [unwired: 10 in, 2 out]
                n302 = Unbundle By Name(w290) -> ("status"=w289:bool)
                n303 = local write "功能逆向初始化"(w289) -> ()
              }
              frame 204 {
                n304 = local read "工位二开始计时"() -> (w308:bool)
                n305 = case shown="假" w308 {
                  tunnel: [w309 _] -> w305
                  frame False {
                    n306 = local read "工位2开始"() -> (w312:u32)
                    n307 = Tick Count (ms)() -> (millisecond timer value=w313:u32)
                    n308 = Subtract(x=w313, y=w312) -> (x-y=w311:u32)
                    n309 = Divide(x=w311, y=u32 1000) -> (x/y=w309:dbl)
                  }
                  frame True {
                    n310 = Tick Count (ms)() -> (millisecond timer value=→"工位2开始":u32)
                    n311 = local write "工位二开始计时"(FALSE ("工位二开始计时")) -> ()
                  }
                }
                n312 = call "传感器数据.vi"() -> ("传感器读数"=w304:T12)  [unwired: 11 in]
                n313 = Unbundle By Name(w304) -> ("2工位压力"=w303:sgl)  [unwired: 1 out]
                n314 = control-ref of="侧铆曲线"() -> (w307:refnum<vi>)
                n315 = call "曲线采集.vi"("曲线引用"=w307, "曲线索引"=0, "X"=w305, "Y"=w303) -> ()  [unwired: 10 in, 2 out]
              }
              frame 300 {
                n316 = local read "工位三开始计时"() -> (w321:bool)
                n317 = case shown="假" w321 {
                  tunnel: [w322 _] -> w318
                  frame False {
                    n318 = local read "工位三开始"() -> (w325:u32)
                    n319 = Tick Count (ms)() -> (millisecond timer value=w326:u32)
                    n320 = Subtract(x=w326, y=w325) -> (x-y=w324:u32)
                    n321 = Divide(x=w324, y=u32 1000) -> (x/y=w322:dbl)
                  }
                  frame True {
                    n322 = Tick Count (ms)() -> (millisecond timer value=→"工位三开始":u32)
                    n323 = local write "工位三开始计时"(FALSE ("工位二开始计时")) -> ()
                  }
                }
                n324 = call "传感器数据.vi"() -> ("传感器读数"=w317:T12)  [unwired: 11 in]
                n325 = Unbundle By Name(w317) -> ("3工位压力"=w316:sgl)  [unwired: 1 out]
                n326 = control-ref of="0°曲线"() -> (w320:refnum<vi>)
                n327 = call "曲线采集.vi"("曲线引用"=w320, "曲线索引"=0, "X"=w318, "Y"=w316) -> ()  [unwired: 10 in, 2 out]
              }
              frame 301 {
                n328 = local read "工位三开始计时1"() -> (w334:bool)
                n329 = case shown="假" w334 {
                  tunnel: [w335 _] -> w331
                  frame False {
                    n330 = local read "工位三开始1"() -> (w338:u32)
                    n331 = Tick Count (ms)() -> (millisecond timer value=w339:u32)
                    n332 = Subtract(x=w339, y=w338) -> (x-y=w337:u32)
                    n333 = Divide(x=w337, y=u32 1000) -> (x/y=w335:dbl)
                  }
                  frame True {
                    n334 = Tick Count (ms)() -> (millisecond timer value=→"工位三开始1":u32)
                    n335 = local write "工位三开始计时1"(FALSE ("工位二开始计时")) -> ()
                  }
                }
                n336 = call "传感器数据.vi"() -> ("传感器读数"=w330:T12)  [unwired: 11 in]
                n337 = Unbundle By Name(w330) -> ("3工位压力"=w329:sgl)  [unwired: 1 out]
                n338 = control-ref of="45°曲线"() -> (w333:refnum<vi>)
                n339 = call "曲线采集.vi"("曲线引用"=w333, "曲线索引"=0, "X"=w331, "Y"=w329) -> ()  [unwired: 10 in, 2 out]
              }
              frame 999 {
                n340 = call "浮动通知.vi"("通知内容"="请启动！" ("Status")) -> ()  [unwired: 11 in]
              }
              frame 1000 {
                n341 = local write "STEP"("扫码" ("STEP")) -> ()
              }
              frame 1002 {
              }
              frame 1024 {
                n342 = local write "STEP"("退出自动" ("STEP")) -> ()
              }
            }
          }
          frame "合格判定" {
            n343 = Wait (ms)(milliseconds to wait=u32 100 ("等待时间（毫秒）")) -> ()  [unwired: 1 out]
            n344 = local write "STEP"("等待" ("STEP")) -> ()
          }
          frame "报表" {
            n345 = stacked-sequence {
              seq-local: [_ w350 _ _] -> [_ _ w355 _]
              frame #0 {
                n346 = global write "Global.vi" "计时开始"(FALSE ("计时开始")) -> ()
                n347 = global read "Global.vi" "产品编号"() -> (w348:string)
                n348 = call "Get_CODE_ID.vi"("CODE_MAIN"=w348) -> ("CODE_ID"=w347:string)  [unwired: 10 in]
                n349 = global write "追溯Global.vi" "CODE_ID"(w347) -> ()
              }
              frame #1 {
                n350 = global read "Global.vi" "产品编号"() -> (w351:string)
                n351 = call "Report.vi"("文件重命名"=TRUE, "文件名称"=w351, "检测结果"="判定结果") -> ("PRODUCT_VAULE"=w350:string)  [unwired: 7 in, 1 out]
              }
              frame #2 {
                n352 = global read "Global.vi" "联机模式"() -> (w354:enum16{"单机", "追溯"})
                n353 = case shown="\"追溯\"" w354 {
                  tunnel: w355 -> [_ w356]
                  frame "单机", Default {
                  }
                  frame "追溯" {
                    n354 = global read "Global.vi" "Result"() -> (w358:refnum<vi>)
                    n355 = property class="Tbl"(reference=w358) -> (reference out=w363:refnum<vi>, error out=w360:errorcluster, "Row Headers[]"=w361:string[])  [unwired: 1 in]
                    n356 = property class="Tbl"(reference=w363, error in=w360) -> (error out=w359:errorcluster, "Value"=w362:string[][])  [unwired: 1 out]
                    n357 = for {
                      tunnel: w362 -> [w370] mode=indexing
                      tunnel: w361 -> [w371] mode=indexing
                      tunnel: [w368] -> w357 mode=indexing if=w369
                      shift-right: [w367] -> _
                      shift-left: w359 -> [w367]
                      n358 = Build Array (concatenate)(w371, w370) -> (w368:string[])
                      n359 = Index Array(array=w370) -> (element=w372:string)  [unwired: 1 in]
                      n360 = case shown="\"\"" w372 {
                        tunnel: [TRUE FALSE] -> w369
                        frame Default {
                        }
                        frame "" {
                        }
                      }
                    }
                    n361 = global read "追溯Global.vi" "DEVICE_ID"() -> (w365:string)
                    n362 = global read "追溯Global.vi" "CODE_ID"() -> (w366:string)
                    n363 = global read "追溯Global.vi" "USER_ID"() -> (w364:string)
                    n364 = call "UPTEST.vi"("Result"=w357, "CODE_ID"=w366, "DEVICE_ID"=w365) -> ()  [unwired: 6 in, 1 out]
                    n365 = call "UPRESULT.vi"("DEVICE_ID"=w365, "USER_ID"=w364, "CODE_ID"=w366, "RESULT_VALUE"=w356) -> ()  [unwired: 11 in, 1 out]
                  }
                }
              }
              frame #3 {
                n366 = local write "STEP"("进入自动" ("STEP")) -> ()
                n367 = global read "检测结果.vi" "合格状态"() -> (w377:string)
                n368 = case shown="\"合格\"" w377 {
                  frame "假", Default {
                  }
                  frame "合格" {
                    n369 = global read "Global.vi" "合格数量"() -> (w380:i32)
                    n370 = Increment(x=w380) -> (x+1=w379:i32)
                    n371 = global write "Global.vi" "合格数量"(w379) -> ()
                  }
                }
                n372 = call "设备状态.vi"("枚举"=enum16{"Read", "Write"}."Write", "Status_Write"=u16 1000 ("设备状态")) -> ()  [unwired: 9 in, 1 out]
              }
            }
          }
        }
        n373 = global read "Global.vi" "程序关闭"() -> (w27:bool)
      }
    }
  }
  n374 = Unregister For Events(event registration refnum=w5) -> ()  [unwired: 1 in, 1 out]
